vi "Calc_DiffR (SubVI).vi"(10 "input valid in":bool, 11 "Mag 3":fxp<+,16,14>) -> (1 "Mag 1":fxp<+,16,14>, 2 "Mag 2":fxp<+,16,14>, 3 "Mag 4":fxp<+,16,14>, 4 "input valid out":bool)   [LabVIEW 2025]
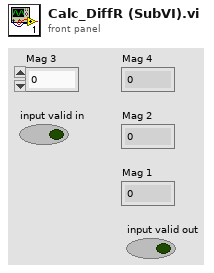
[diagram p1: front panel]
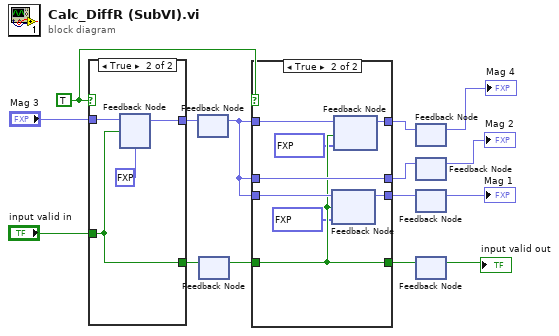
[diagram p0: block diagram]
diagram:
  w12 = TRUE
  n1 = case shown="True" w12 {
    tunnel: [w17 w20] -> w15
    tunnel: "input valid in" -> [w16 w19]
    tunnel: [w16 w19] -> w13
    tunnel: "Mag 3" -> [w17 w21]
    frame False {
    }
    frame True {
      n2 = feedback #1(fxp<+,16,14> 0.0 ("Mag 3")) -> (w20:fxp<+,16,14>)
      n3 = feedback-in #1(w21, w19) -> ()
    }
  }
  n4 = feedback #2() -> (w1:fxp<+,16,14>)  [unwired: 1 in]
  n5 = feedback-in #2(w15) -> ()
  n6 = feedback #3() -> (w14:bool)  [unwired: 1 in]
  n7 = feedback-in #3(w13) -> ()
  n8 = case shown="True" w12 {
    tunnel: w1 -> [w25 w30]
    tunnel: [w25 w29] -> w9
    tunnel: w1 -> [w23 w32]
    tunnel: [w23 w31] -> w5
    tunnel: w14 -> [w22 w28]
    tunnel: [w22 w28] -> w3
    tunnel: w1 -> [w24 w33]
    tunnel: [w24 w33] -> w7
    frame False {
    }
    frame True {
      n9 = feedback #4(fxp<+,16,14>[] [0.0, 0.0, 0.0, 0.0, 0.0, 0.0, 0.0, 0.0, 0.0, 0.0, 0.0, 0.0, 0.0, 0.0, 0.0, 0.0, 0.0, 0.0, 0.0, 0.0, 0.0, 0.0, 0.0, 0.0, 0.0, 0.0, 0.0, 0.0, 0.0, 0.0, 0.0, 0.0, 0.0, 0.0, 0.0, 0.0, 0.0, 0.0, 0.0, 0.0, 0.0, 0.0, 0.0, 0.0, 0.0, 0.0, 0.0, 0.0, 0.0, 0.0, 0.0, 0.0, 0.0, 0.0, 0.0, 0.0, 0.0, 0.0, 0.0, 0.0, 0.0, 0.0, 0.0, 0.0]) -> (w31:fxp<+,16,14>)
      n10 = feedback-in #4(w32, w28) -> ()
      n11 = feedback #5(fxp<+,16,14>[] [0.0, 0.0, 0.0, 0.0, 0.0, 0.0, 0.0, 0.0, 0.0, 0.0, 0.0, 0.0, 0.0, 0.0, 0.0, 0.0, 0.0, 0.0, 0.0, 0.0, 0.0, 0.0, 0.0, 0.0, 0.0, 0.0, 0.0, 0.0, 0.0, 0.0, 0.0, 0.0]) -> (w29:fxp<+,16,14>)
      n12 = feedback-in #5(w30, w28) -> ()
    }
  }
  n13 = feedback #6() -> (→"Mag 4":fxp<+,16,14>)  [unwired: 1 in]
  n14 = feedback-in #6(w9) -> ()
  n15 = feedback #7() -> (→"Mag 2":fxp<+,16,14>)  [unwired: 1 in]
  n16 = feedback-in #7(w7) -> ()
  n17 = feedback #8() -> (→"Mag 1":fxp<+,16,14>)  [unwired: 1 in]
  n18 = feedback-in #8(w5) -> ()
  n19 = feedback #9() -> (→"input valid out":bool)  [unwired: 1 in]
  n20 = feedback-in #9(w3) -> ()
